vi "Image Viewer.vi"(9 "Stop":bool, 10 "List of Image Files":i32(listbox), 11 "Folder Path":path) -> (2 "2D Picture":picture, 3 "Message BOX":string)   [LabVIEW 2020]
doc: "This VI will load user selected folder containing Image files and will display the selected image on the 2D Picture Display."
uses:
  <vilib>/picture/picture.llb/imagedata.ctl
  <vilib>/Utility/miscctls.llb/LVBoundsTypeDef.ctl
panel:
  in  "OK":bool
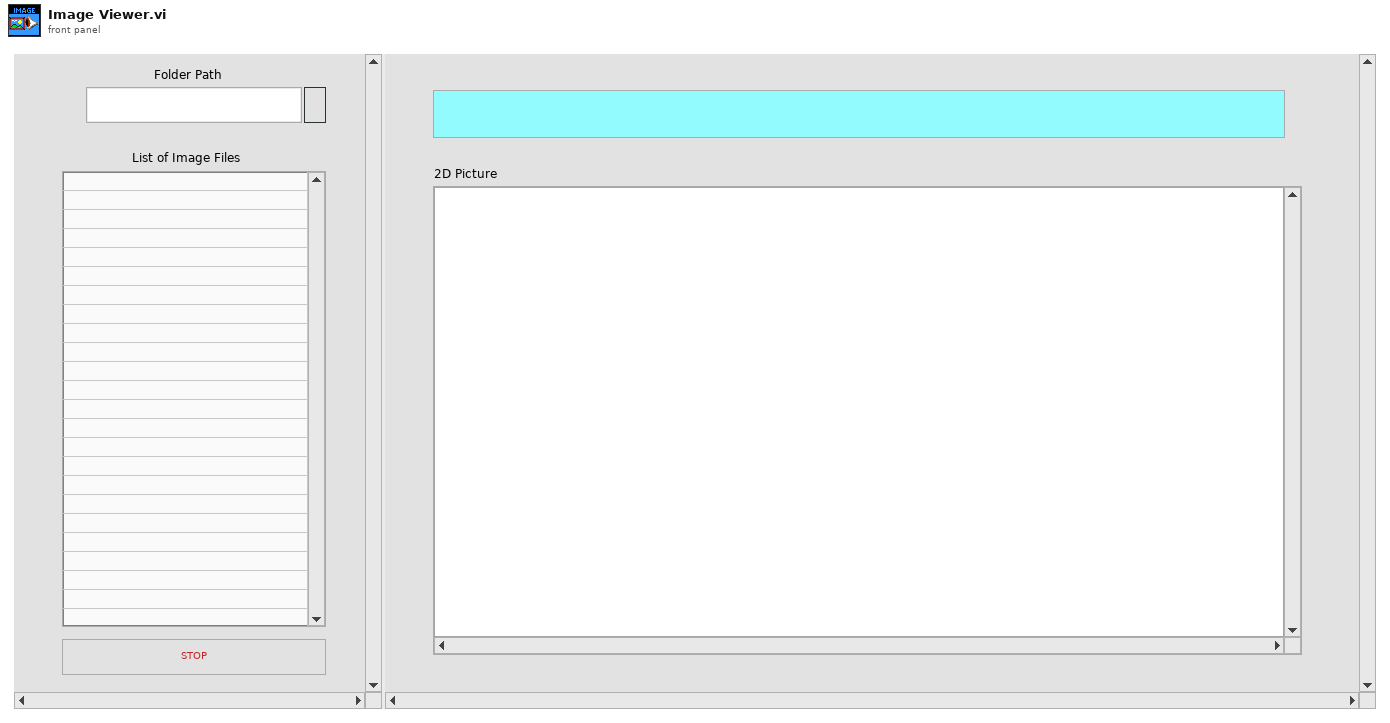
[diagram p1: front panel]
types:
  T1 = enum32{"Invalid", "Standard", "Closed", "Hidden", "Minimized", "Maximized"}
  T2 = enum32{"invalid app kind", "Development System", "Run Time System", "Student Edition", "Embedded LabVIEW", "Evaluation", "Custom"}
  T3 = typedef "LVBoundsTypeDef.ctl" = cluster{"Width":u32, "Height":u32}
  T4 = typedef "imagedata.ctl" = cluster{"image type":i32, "image depth":i32, "image":u8[], "mask":u8[], "colors":u32[], "Rectangle":cluster{"left":i16, "top":i16, "right":i16, "bottom":i16}}
  T5 = cluster{"Core":cluster{"Current VI Reference":refnum<vi>, "Close Panel on Exit?":bool}, "Your Boolean data":bool, "Message BOX":string, "Folder Path":path, "File Name":string, " picture":picture, "image data":T4}
  T6 = cluster{"Current VI Reference":refnum<vi>, "Close Panel on Exit?":bool}
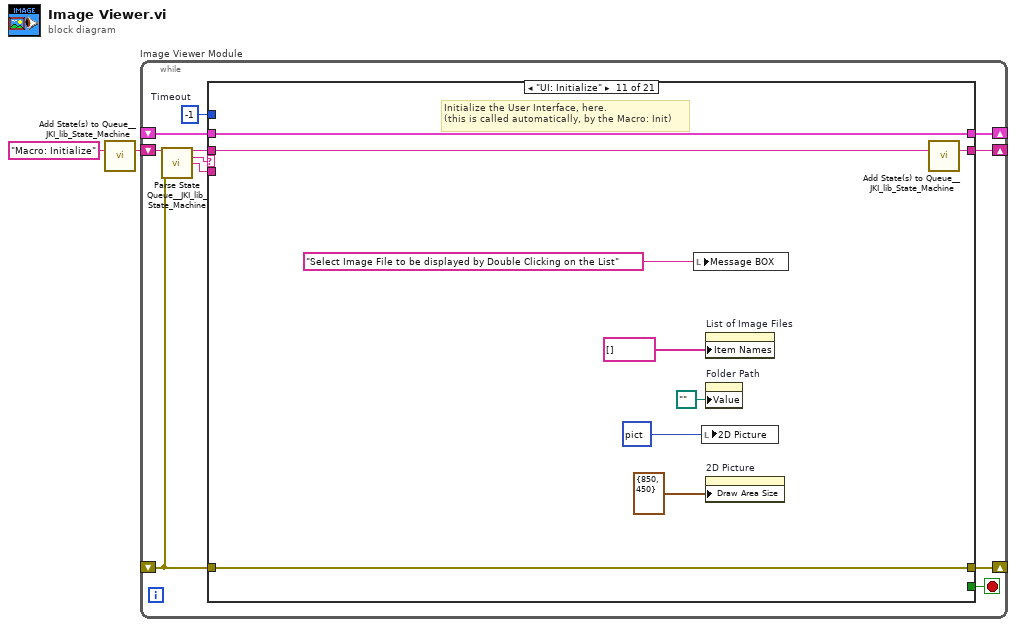
[diagram p0: block diagram]
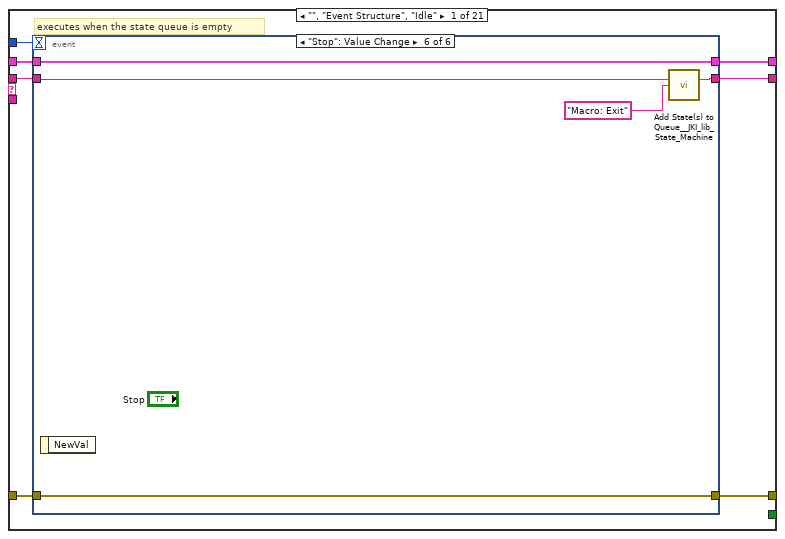
[diagram p2: hidden frame]
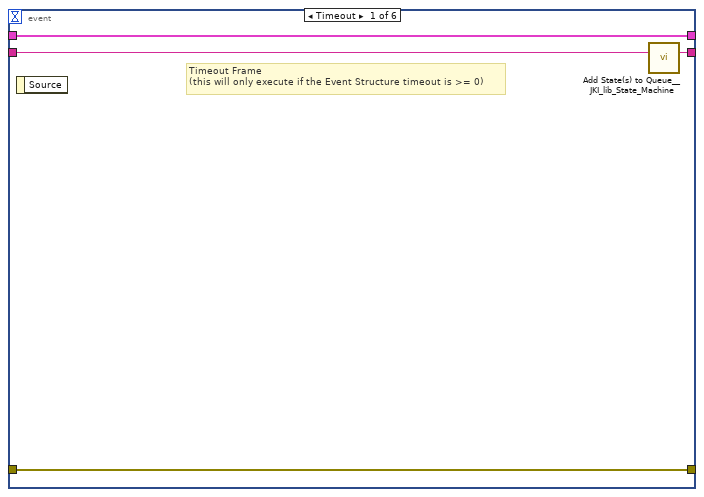
[diagram p3: hidden frame]
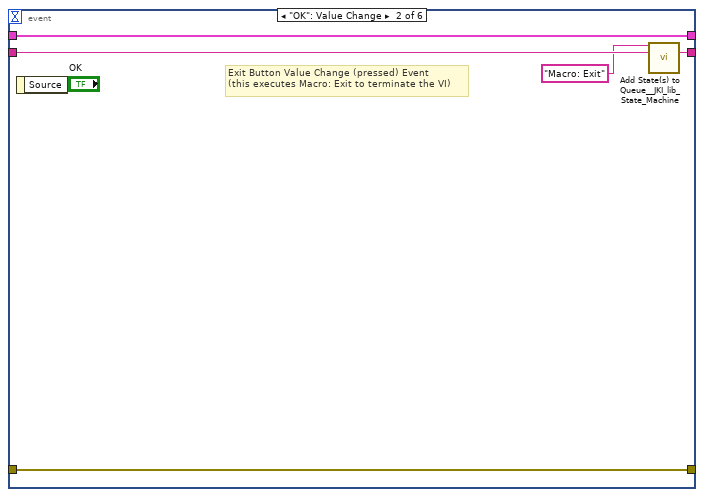
[diagram p4: hidden frame]
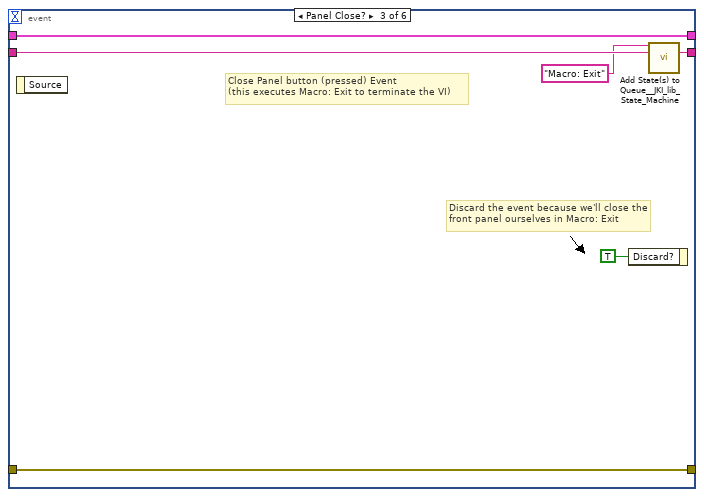
[diagram p5: hidden frame]
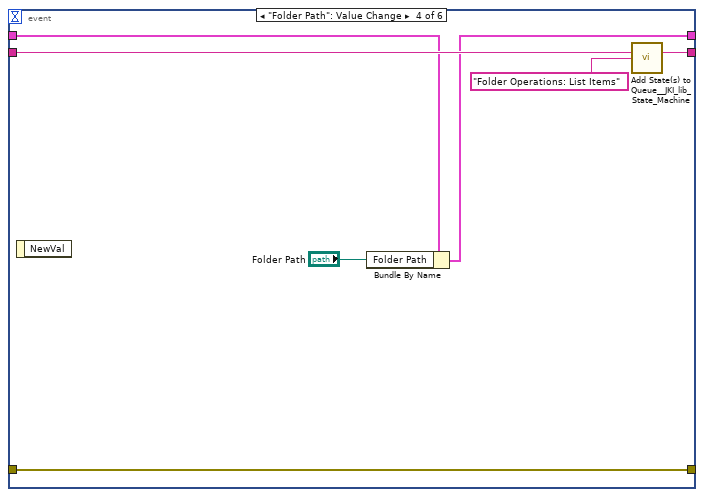
[diagram p6: hidden frame]
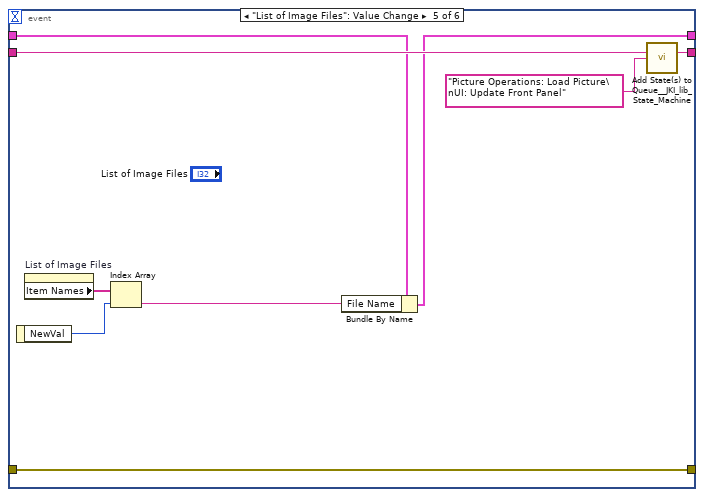
[diagram p7: hidden frame]
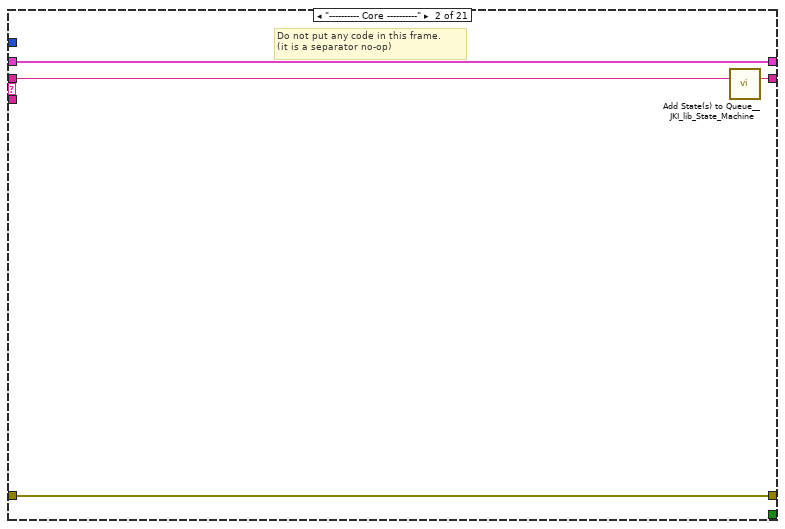
[diagram p8: hidden frame]
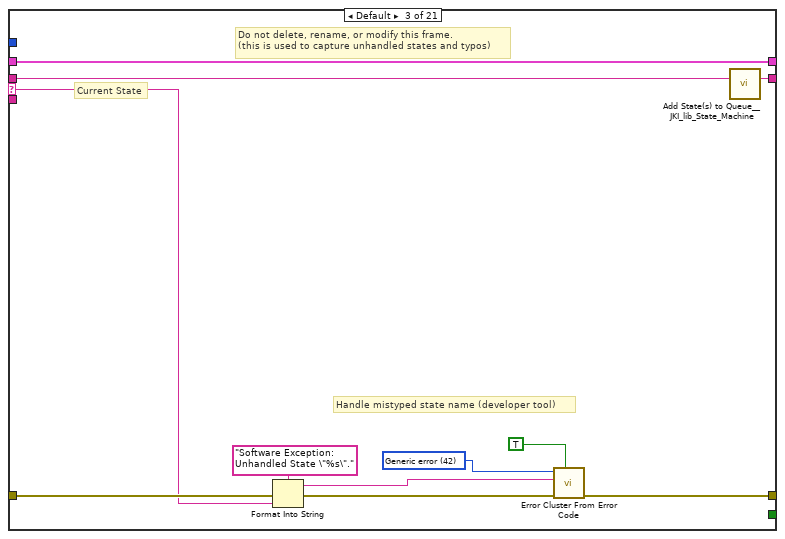
[diagram p9: hidden frame]
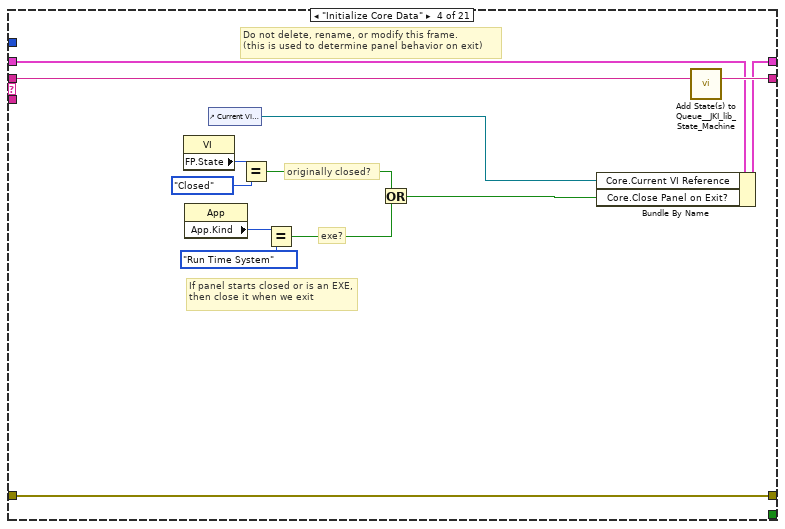
[diagram p10: hidden frame]
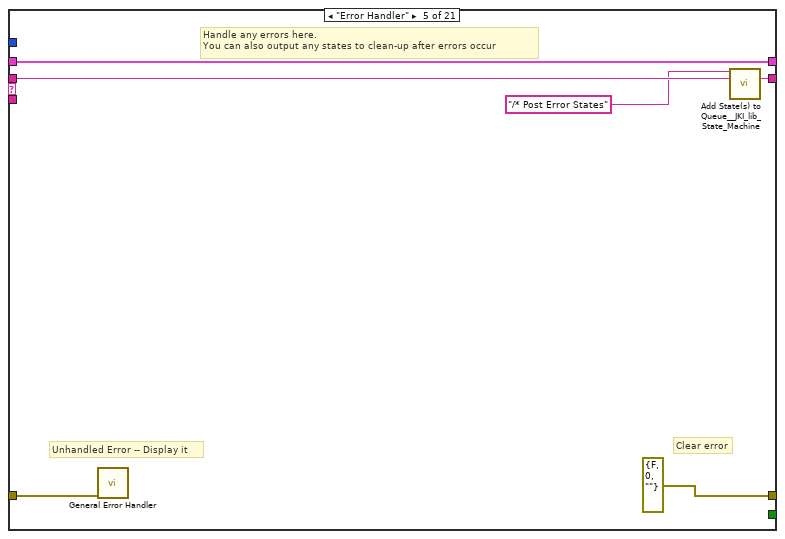
[diagram p11: hidden frame]
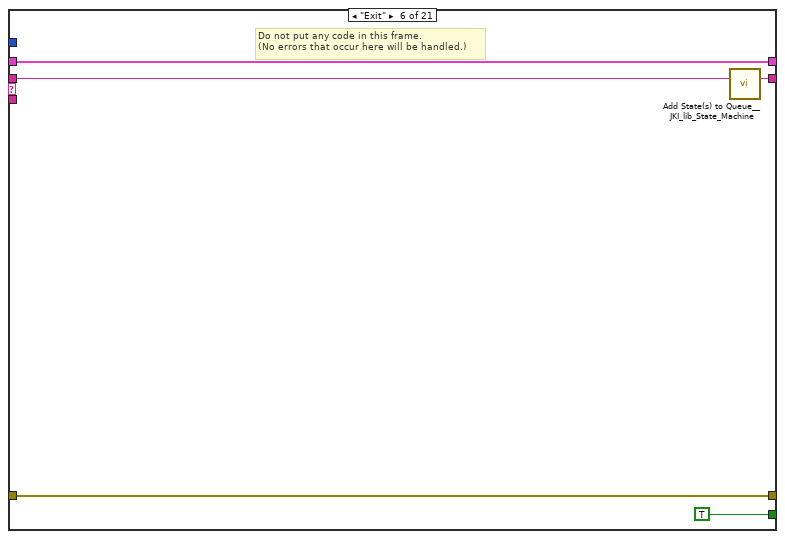
[diagram p12: hidden frame]
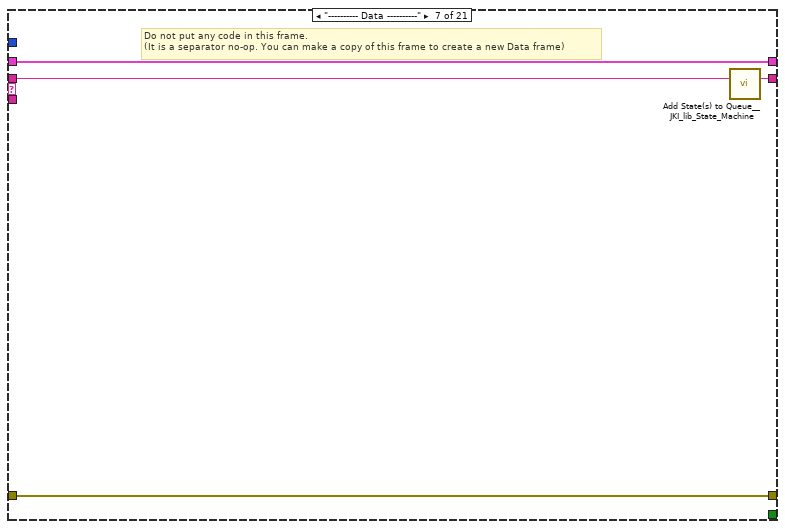
[diagram p13: hidden frame]
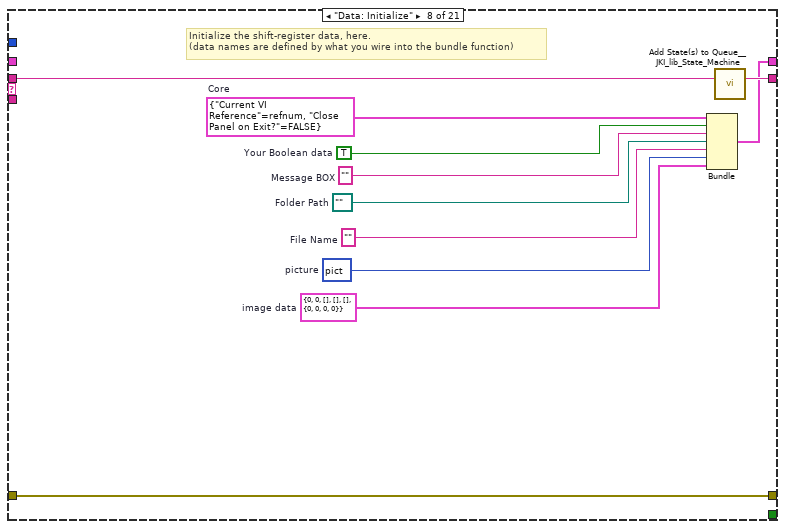
[diagram p14: hidden frame]
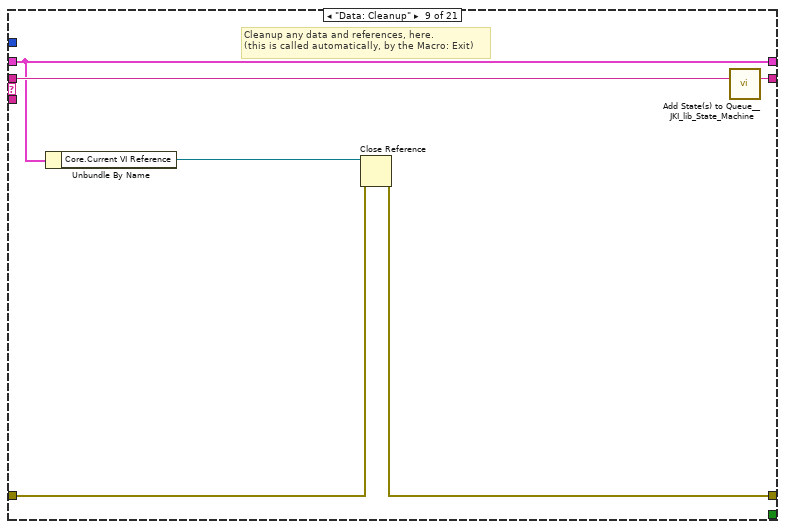
[diagram p15: hidden frame]
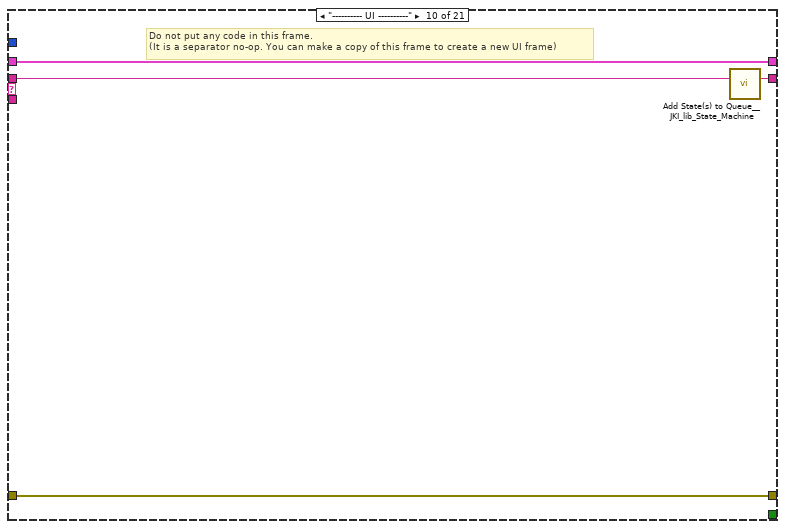
[diagram p16: hidden frame]
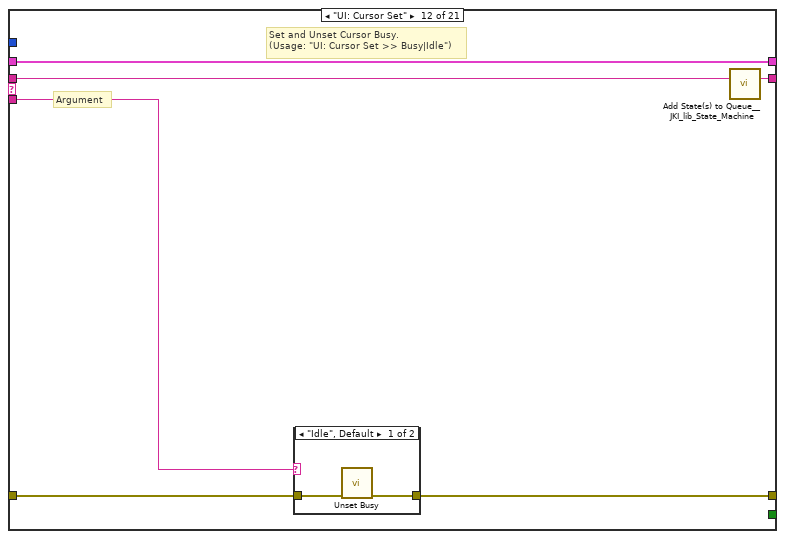
[diagram p17: hidden frame]
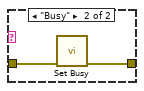
[diagram p18: hidden frame]
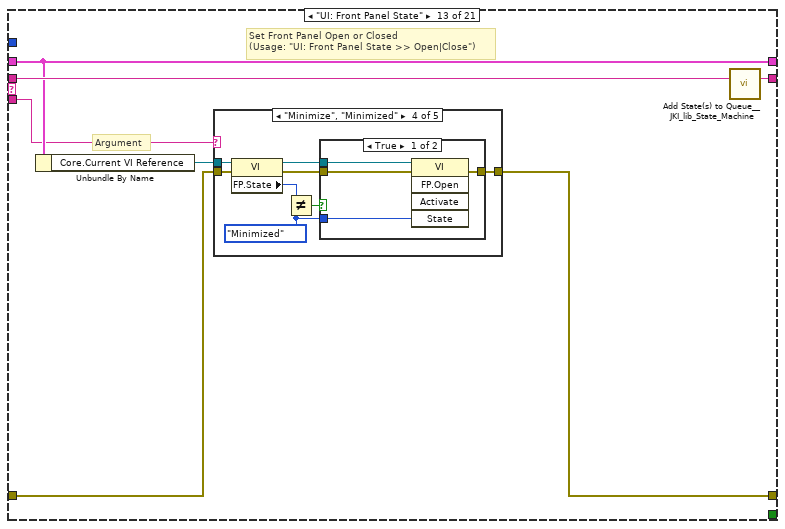
[diagram p19: hidden frame]
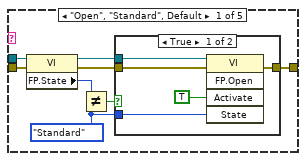
[diagram p20: hidden frame]
diagram:
  n1 = call <vilib>:"Add State(s) to Queue__JKI_lib_State_Machine.vi"("State(s) in (\"\")"="Macro: Initialize") -> ("States Out"=w2:string)  [unwired: 14 in]
  n2 = while "Image Viewer Module" {
    shift-right: [w6] -> _
    shift-left: _ -> [w5]
    shift-right: [w9] -> _
    shift-left: _ -> [w3]
    shift-right: [w8] -> _
    shift-left: w2 -> [w10]
    stop <- w7 stop-if-true
    w4 = -1  # Timeout
    n3 = call <vilib>:"Parse State Queue__JKI_lib_State_Machine.vi"("State Queue"=w10, "Error In (no error)"=w3) -> ("Remaining States"=w12:string, "Current State"=w13:string, "Arguments"=w11:string)  [unwired: 11 in]
    n4 = case shown="\"UI: Initialize\"" w13 {
      selector: w13 -> [_ _ w61 _ _ _ _ _ _ _ _ _ _ _ _ _ _ _ _ _ _]
      tunnel: w12 -> [w20 w60 w65 w84 w90 w95 w99 w110 w116 w120 w129 w135 w146 w224 w228 w233 w243 w247 w253 w257 w274]
      tunnel: w11 -> [_ _ _ _ _ _ _ _ _ _ _ w130 w140 _ _ _ _ _ _ _ _]
      tunnel: w5 -> [w18 w57 w63 w77 w87 w93 w96 _ w111 w117 w127 w133 w142 w221 w225 w230 w240 w244 w250 w254 w268]
      tunnel: [w17 w58 w67 w81 errorcluster {"status"=FALSE, "code"=0, "source"=""} ("error out") w92 w97 w107 w112 w118 w126 w131 w143 w222 w226 w231 w241 w245 w251 w255 w272] -> w9
      tunnel: w3 -> [w16 w58 w66 w81 w86 w92 w97 w107 w113 w118 w126 w132 w144 w222 w226 w231 w241 w245 w251 w255 w272]
      tunnel: [w19 w59 w64 w83 w89 w94 w98 w109 w115 w119 w128 w134 w145 w223 w227 w232 w242 w246 w252 w256 w273] -> w8
      tunnel: [_ _ _ _ _ TRUE _ _ _ _ _ _ _ _ _ _ _ _ _ _ _] -> w7
      tunnel: [w15 w57 w63 w82 w87 w93 w96 w108 w111 w117 w127 w133 w142 w221 w225 w230 w240 w244 w250 w254 w267] -> w6
      tunnel: w4 -> [w14 _ _ _ _ _ _ _ _ _ _ _ _ _ _ _ _ _ _ _ _]
      frame "", "Event Structure", "Idle" {
        # "executes when the state queue is empty"
        n5 = event shown="[5] \"Stop\": Value Change" {
          selector: _ -> [_ _ _ _ _ _]
          dyn-events: _ -> [_ _ _ _ _ _]
          timeout: w14 -> [_ _ _ _ _ _]
          tunnel: w20 -> [w24 w29 w35 w41 w50 w54]
          tunnel: [w23 w28 w34 w42 w51 w55] -> w19
          tunnel: w18 -> [w21 w26 w32 w40 w46 w53]
          tunnel: [w22 w27 w33 w36 w49 w56] -> w17
          tunnel: w16 -> [w22 w27 w33 w36 w49 w56]
          tunnel: [w21 w26 w32 w39 w45 w53] -> w15
          event Timeout {
            # "Timeout Frame\n(this will only execute if the Event Structure timeout is >= 0)"
            n6 = event-data() -> ()  [unwired: 1 in, 1 out]
            n7 = call <vilib>:"Add State(s) to Queue__JKI_lib_State_Machine.vi"("State(s) in (\"\")"=w24) -> ("States Out"=w23:string)  [unwired: 14 in]
          }
          event "OK": Value Change {
            # "Exit Button Value Change (pressed) Event\n(this executes Macro: Exit to terminate the VI)"
            n8 = event-data() -> ()  [unwired: 1 in, 1 out]
            n9 = call <vilib>:"Add State(s) to Queue__JKI_lib_State_Machine.vi"("State(s) in Front (\"\")"="Macro: Exit", "State(s) in (\"\")"=w29) -> ("States Out"=w28:string)  [unwired: 13 in]
          }
          event Panel Close? {
            # "Discard the event because we'll close the front panel ourselves in Macro: Exit"
            # "Close Panel button (pressed) Event\n(this executes Macro: Exit to terminate the VI)"
            n10 = event-data() -> ()  [unwired: 1 in, 1 out]
            n11 = event-data("Discard?"=TRUE) -> ()  [unwired: 1 in, 1 out]
            n12 = call <vilib>:"Add State(s) to Queue__JKI_lib_State_Machine.vi"("State(s) in Front (\"\")"="Macro: Exit", "State(s) in (\"\")"=w35) -> ("States Out"=w34:string)  [unwired: 13 in]
          }
          event "Folder Path": Value Change {
            n13 = event-data() -> ()  [unwired: 1 in, 1 out]
            n14 = Bundle By Name(cluster=w40, "Folder Path"="Folder Path") -> (w39:T5)
            n15 = call <vilib>:"Add State(s) to Queue__JKI_lib_State_Machine.vi"("State(s) in (\"\")"=w41, "State(s) at Back (\"\")"="Folder Operations: List Items" ("State(s) at Back (\"\")")) -> ("States Out"=w42:string)  [unwired: 13 in]
          }
          event "List of Image Files": Value Change {
            n16 = event-data() -> ("NewVal"=w47:i32)  [unwired: 1 in]
            n17 = property on="List of Image Files" class="LstBox (strict)"() -> ("Item Names"=w48:string[])  [unwired: 2 in, 2 out]
            n18 = Index Array(array=w48, index=w47) -> (element=w44:string)
            n19 = Bundle By Name(cluster=w46, "File Name"=w44) -> (w45:T5)
            n20 = call <vilib>:"Add State(s) to Queue__JKI_lib_State_Machine.vi"("State(s) in (\"\")"=w50, "State(s) at Back (\"\")"="Picture Operations: Load Picture\nUI: Update Front Panel" ("State(s) at Back (\"\")")) -> ("States Out"=w51:string)  [unwired: 13 in]
          }
          event "Stop": Value Change {
            n21 = event-data() -> ()  [unwired: 1 in, 1 out]
            n22 = call <vilib>:"Add State(s) to Queue__JKI_lib_State_Machine.vi"("State(s) in (\"\")"=w54, "State(s) at Back (\"\")"="Macro: Exit") -> ("States Out"=w55:string)  [unwired: 13 in]
          }
        }
      }
      frame "---------- Core ----------" {
        # "Do not put any code in this frame.\n(it is a separator no-op)"
        n23 = call <vilib>:"Add State(s) to Queue__JKI_lib_State_Machine.vi"("State(s) in (\"\")"=w60) -> ("States Out"=w59:string)  [unwired: 14 in]
      }
      frame Default {
        w70 = 42 items=["No error", "Argument error", "Memory is full", "Out of zone", "End of file", "File already open", "Generic file I/O error", "File not found", "File permission error", "Disk is full", "Duplicate path", "Too many files open", "System feature not enabled", "Resource file not found", "Cannot add resource", "Resource not found", "Image not found", "Image memory error", "Pen does not exist", "Config type invalid", "Config token not found", "Config parse error", "Config memory error", "Bad external code format", "Bad external code offset", "External code not present", "Null window", "Destroy window error", "Null menu", "Print aborted", "Bad print record", "Print driver error", "Windows error during printing", "Memory error during printing", "Print dialog error", "Generic print error", "Invalid device refnum", "Device not found", "Device parameter error", "Device unit error", "Cannot open device", "Device call aborted", "Generic error", "Cancelled by user", "Object ID too low", "Object ID too high", "Object not in heap", "Unknown heap", "Unknown object (invalid DefProc)", "Unknown object (DefProc not in table)", "Message out of range", "Invalid (null) method", "Unknown message", "Manager call not supported", "Bad address", "Network operation in progress", "Network operation timed out", "Connection is busy", "Network attribute not supported", "Network error", "Address in use", "System out of memory", "Connection aborted", "Connection refused", "Not connected", "Already connected", "Connection closed", "Initialization error (interapplication manager)", "Bad occurrence", "Wait on unbound occurrence handler", "Occurrence queue overflow", "Datalog type conflict", "Unused", "Unrecognized type (interapplication manager)", "Memory corrupt", "Failed to make temporary DLL", "Old CIN version", "Drag socket not found", "Failed to load drop-object", "Failed to register OLE object", "Failed to release OLE object", "Format specifier type mismatch", "Unknown format specifier", "Too few format specifiers", "Too many format specifiers", "Scan failed", "Newer CIN version", "Error converting to variant", "Runtime menu error", "Password tampered", "Variant attribute not found", "Incompatible variant data type", "Event data is not available", "Event Store is not present", "Occurrence is not found", "Event Queue is not created", "Event info is not available", "Refnum passed is NULL", "Error retrieving Class GUID", "Error retrieving CoClass GUID", "Error retrieving TypeLib GUID.", "Bad built application magic bytes.", "Specific driver is different from the specific driver associated with the Logical Name.", "There is no session opened to the class driver.", "Max Error", "MAX - Error with config objects", "MAX - Error loading configuration", "MAX - Group not supported"]
        # "Current State"
        # "Do not delete, rename, or modify this frame.\n(this is used to capture unhandled states and typos)"
        # "Handle mistyped state name (developer tool)"
        n24 = Format Into String(format string="Software Exception: Unhandled State \"%s\"." ("message"), error in=w66, w61) -> (resulting string=w69:string, error out=w68:errorcluster)  [unwired: 1 in]
        n25 = call <vilib>:"Error Cluster From Error Code.vi"("show call chain? (False)"=TRUE, "error in (no error)"=w68, "error message (\"\")"=w69, "error code (0)"=w70) -> ("error out"=w67:errorcluster)  [unwired: 5 in]
        n26 = call <vilib>:"Add State(s) to Queue__JKI_lib_State_Machine.vi"("State(s) in (\"\")"=w65) -> ("States Out"=w64:string)  [unwired: 14 in]
      }
      frame "Initialize Core Data" {
        # "Do not delete, rename, or modify this frame.\n(this is used to determine panel behavior on exit)"
        # "originally closed?"
        # "exe?"
        # "If panel starts closed or is an EXE, then close it when we exit"
        n27 = property class="VI"() -> ("FP.State"=w74:T1)  [unwired: 2 in, 2 out]
        n28 = property class="App"() -> ("App.Kind"=w80:T2)  [unwired: 2 in, 2 out]
        n29 = control-ref of="Current VI Reference"() -> (w75:refnum<vi>)
        n30 = Equal?(x=w74, y=T1."Closed" ("Front Panel Window:State")) -> (x = y?=w72:bool)
        n31 = Equal?(x=w80, y=T2."Run Time System" ("Application:Kind")) -> (x = y?=w78:bool)
        n32 = Or(x=w72, y=w78) -> (x .or. y?=w76:bool)
        n33 = Bundle By Name(cluster=w77, "Core.Current VI Reference"=w75, "Core.Close Panel on Exit?"=w76) -> (w82:T5)
        n34 = call <vilib>:"Add State(s) to Queue__JKI_lib_State_Machine.vi"("State(s) in (\"\")"=w84) -> ("States Out"=w83:string)  [unwired: 14 in]
      }
      frame "Error Handler" {
        # "Unhandled Error -- Display it"
        # "Handle any errors here.\nYou can also output any states to clean-up after errors occur"
        # "Clear error"
        n35 = call <vilib>:"General Error Handler.vi"("error in (no error)"=w86) -> ()  [unwired: 10 in, 5 out]
        n36 = call <vilib>:"Add State(s) to Queue__JKI_lib_State_Machine.vi"("State(s) in Front (\"\")"="/* Post Error States", "State(s) in (\"\")"=w90) -> ("States Out"=w89:string)  [unwired: 13 in]
      }
      frame "Exit" {
        # "Do not put any code in this frame.\n(No errors that occur here will be handled.)"
        n37 = call <vilib>:"Add State(s) to Queue__JKI_lib_State_Machine.vi"("State(s) in (\"\")"=w95) -> ("States Out"=w94:string)  [unwired: 14 in]
      }
      frame "---------- Data ----------" {
        # "Do not put any code in this frame.\n(It is a separator no-op. You can make a copy of this frame to create a new Data frame)"
        n38 = call <vilib>:"Add State(s) to Queue__JKI_lib_State_Machine.vi"("State(s) in (\"\")"=w99) -> ("States Out"=w98:string)  [unwired: 14 in]
      }
      frame "Data: Initialize" {
        w100 = T4 {"image type"=0, "image depth"=0, "image"=[], "mask"=[], "colors"=[], "Rectangle"={"left"=0, "top"=0, "right"=0, "bottom"=0}}  # image data
        w101 = picture data[5B]  # picture
        w102 = ""  # File Name
        w103 = path ""  # Folder Path
        w104 = T6 {"Current VI Reference"=refnum, "Close Panel on Exit?"=FALSE}  # Core
        w106 = TRUE  # Your Boolean data
        w105 = ""  # Message BOX
        # "Initialize the shift-register data, here.\n(data names are defined by what you wire into the bundle function)"
        n39 = Bundle("Core"=w104, "Your Boolean data"=w106, "Message BOX"=w105, "Folder Path"=w103, "File Name"=w102, "picture"=w101, "image data"=w100) -> (w108:T5)  [unwired: 1 in]
        n40 = call <vilib>:"Add State(s) to Queue__JKI_lib_State_Machine.vi"("State(s) in (\"\")"=w110) -> ("States Out"=w109:string)  [unwired: 14 in]
      }
      frame "Data: Cleanup" {
        # "Cleanup any data and references, here.\n(this is called automatically, by the Macro: Exit)"
        n41 = Unbundle By Name(w111) -> ("Core.Current VI Reference"=w114:refnum<vi>)
        n42 = Close Reference(reference=w114, error in (no error)=w113) -> (error out=w112:errorcluster)
        n43 = call <vilib>:"Add State(s) to Queue__JKI_lib_State_Machine.vi"("State(s) in (\"\")"=w116) -> ("States Out"=w115:string)  [unwired: 14 in]
      }
      frame "---------- UI ----------" {
        # "Do not put any code in this frame.\n(It is a separator no-op. You can make a copy of this frame to create a new UI frame)"
        n44 = call <vilib>:"Add State(s) to Queue__JKI_lib_State_Machine.vi"("State(s) in (\"\")"=w120) -> ("States Out"=w119:string)  [unwired: 14 in]
      }
      frame "UI: Initialize" {
        # "Initialize the User Interface, here.\n(this is called automatically, by the Macro: Init)"
        n45 = local write "Message BOX"("Select Image File to be displayed by Double Clicking on the List" ("Message BOX")) -> ()
        n46 = local write "2D Picture"(picture data[5B] ("2D Picture")) -> ()
        n47 = property on="List of Image Files" class="LstBox (strict)"("Item Names"=string[] []) -> ()  [unwired: 2 in, 2 out]
        n48 = property on="Folder Path" class="Path"("Value"=path "" ("Folder Path")) -> ()  [unwired: 2 in, 2 out]
        n49 = property on="2D Picture" class="Pict"("Draw Area Size"=T3 {"Width"=850, "Height"=450}) -> ()  [unwired: 2 in, 2 out]
        n50 = call <vilib>:"Add State(s) to Queue__JKI_lib_State_Machine.vi"("State(s) in (\"\")"=w129) -> ("States Out"=w128:string)  [unwired: 14 in]
      }
      frame "UI: Cursor Set" {
        # "Argument"
        # "Set and Unset Cursor Busy.\n(Usage: \"UI: Cursor Set >> Busy|Idle\")"
        n51 = case shown="\"Idle\", Default" w130 {
          tunnel: w132 -> [w137 w139]
          tunnel: [w136 w138] -> w131
          frame "Idle", Default {
            n52 = call <vilib>:"Unset Busy.vi"("error in (no error)"=w137) -> ("error out"=w136:errorcluster)  [unwired: 10 in]
          }
          frame "Busy" {
            n53 = call <vilib>:"Set Busy.vi"("error in (no error)"=w139) -> ("error out"=w138:errorcluster)  [unwired: 9 in, 1 out]
          }
        }
        n54 = call <vilib>:"Add State(s) to Queue__JKI_lib_State_Machine.vi"("State(s) in (\"\")"=w135) -> ("States Out"=w134:string)  [unwired: 14 in]
      }
      frame "UI: Front Panel State" {
        # "Argument"
        # "Set Front Panel Open or Closed\n(Usage: \"UI: Front Panel State >> Open|Close\")"
        n55 = Unbundle By Name(w142) -> ("Core.Current VI Reference"=w141:refnum<vi>)
        n56 = case shown="\"Minimize\", \"Minimized\"" w140 {
          tunnel: w144 -> [w152 w167 w178 w191 w204]
          tunnel: [w154 w168 w180 w193 w206] -> w143
          tunnel: w141 -> [w153 w165 w179 w192 w205]
          frame "Open", "Standard", Default {
            w147 = T1."Standard" ("State")
            n57 = property class="VI"(reference=w153, error in=w152) -> (reference out=w150:refnum<vi>, error out=w151:errorcluster, "FP.State"=w149:T1)
            n58 = Not Equal?(x=w149, y=w147) -> (x != y?=w148:bool)
            n59 = case shown="True" w148 {
              tunnel: [w158 w160] -> w154
              tunnel: w151 -> [w157 w160]
              tunnel: w150 -> [w156 _]
              tunnel: w147 -> [w155 _]
              frame True {
                n60 = invoke class="VI" method="FP.Open"(reference=w156, error in=w157, "Activate"=TRUE, "State"=w155) -> (error out=w158:errorcluster)  [unwired: 1 in, 4 out]
              }
              frame False {
              }
            }
          }
          frame "Close", "Closed" {
            n61 = property class="VI"(reference=w165, error in=w167) -> (reference out=w164:refnum<vi>, error out=w166:errorcluster, "FP.State"=w162:T1)
            n62 = Not Equal?(x=w162, y=T1."Closed" ("Front Panel Window:State")) -> (x != y?=w161:bool)
            n63 = case shown="True" w161 {
              tunnel: [w169 w172] -> w168
              tunnel: w166 -> [w169 w171]
              tunnel: w164 -> [_ w170]
              frame False {
              }
              frame True {
                n64 = invoke class="VI" method="FP.Close"(reference=w170, error in=w171) -> (error out=w172:errorcluster)  [unwired: 1 in, 2 out]
              }
            }
          }
          frame "Hidden", "Hide" {
            w173 = T1."Hidden" ("State")
            n65 = property class="VI"(reference=w179, error in=w178) -> (reference out=w176:refnum<vi>, error out=w177:errorcluster, "FP.State"=w175:T1)
            n66 = Not Equal?(x=w175, y=w173) -> (x != y?=w174:bool)
            n67 = case shown="True" w174 {
              tunnel: [w184 w185] -> w180
              tunnel: w177 -> [w183 w185]
              tunnel: w176 -> [w182 _]
              tunnel: w173 -> [w181 _]
              frame True {
                n68 = invoke class="VI" method="FP.Open"(reference=w182, error in=w183, "State"=w181) -> (error out=w184:errorcluster)  [unwired: 2 in, 4 out]
              }
              frame False {
              }
            }
          }
          frame "Minimize", "Minimized" {
            w186 = T1."Minimized" ("State")
            n69 = property class="VI"(reference=w192, error in=w191) -> (reference out=w189:refnum<vi>, error out=w190:errorcluster, "FP.State"=w188:T1)
            n70 = Not Equal?(x=w188, y=w186) -> (x != y?=w187:bool)
            n71 = case shown="True" w187 {
              tunnel: [w197 w198] -> w193
              tunnel: w190 -> [w196 w198]
              tunnel: w189 -> [w195 _]
              tunnel: w186 -> [w194 _]
              frame True {
                n72 = invoke class="VI" method="FP.Open"(reference=w195, error in=w196, "State"=w194) -> (error out=w197:errorcluster)  [unwired: 2 in, 4 out]
              }
              frame False {
              }
            }
          }
          frame "Maximize", "Maximized" {
            w199 = T1."Maximized" ("State")
            n73 = property class="VI"(reference=w205, error in=w204) -> (reference out=w202:refnum<vi>, error out=w203:errorcluster, "FP.State"=w201:T1)
            n74 = Not Equal?(x=w201, y=w199) -> (x != y?=w200:bool)
            n75 = case shown="True" w200 {
              tunnel: [w210 w211] -> w206
              tunnel: w203 -> [w209 w211]
              tunnel: w202 -> [w208 _]
              tunnel: w199 -> [w207 _]
              frame True {
                n76 = invoke class="VI" method="FP.Open"(reference=w208, error in=w209, "State"=w207) -> (error out=w210:errorcluster)  [unwired: 2 in, 4 out]
              }
              frame False {
              }
            }
          }
        }
        n77 = call <vilib>:"Add State(s) to Queue__JKI_lib_State_Machine.vi"("State(s) in (\"\")"=w146) -> ("States Out"=w145:string)  [unwired: 14 in]
      }
      frame "UI: Update Front Panel" {
        # "Front Panel update based on USER input\n(Updates Front Panel 2D Picture Box with the Image)"
        n78 = Unbundle By Name(w221) -> ("File Name"=w220:string, "image data"=w217:T4, "picture"=→"2D Picture":picture)
        n79 = Concatenate Strings("You have Selected " ("string"), w220) -> (→"Message BOX":string)
        n80 = Unbundle By Name(w217) -> ("Rectangle.right"=w216:i16, "Rectangle.bottom"=w215:i16)
        n81 = Bundle(cluster=cluster{"right":i16, "bottom":i16} {"right"=0, "bottom"=0}, "right"=w216, "bottom"=w215) -> (w213:cluster{"right":i16, "bottom":i16})
        n82 = property on="2D Picture" class="Pict"("Draw Area Size"=w213) -> ()  [unwired: 2 in, 2 out]
        n83 = call <vilib>:"Add State(s) to Queue__JKI_lib_State_Machine.vi"("State(s) in (\"\")"=w224) -> ("States Out"=w223:string)  [unwired: 14 in]
      }
      frame "---------- Macro ----------" {
        # "Do not put any code in this frame.\n(It is a separator no-op. You can make a copy of this frame to create a new Macro frame)"
        n84 = call <vilib>:"Add State(s) to Queue__JKI_lib_State_Machine.vi"("State(s) in (\"\")"=w228) -> ("States Out"=w227:string)  [unwired: 14 in]
      }
      frame "Macro: Initialize" {
        w229 = "Data: Initialize\nInitialize Core Data\nUI: Initialize\nUI: Front Panel State >> Open"  # Data: Initialize Initialize Core Data UI: Initialize UI: Front Panel State >> Open
        # "Initialization Macro\n(This is called once, when the VI starts)"
        n85 = call <vilib>:"Add State(s) to Queue__JKI_lib_State_Machine.vi"("State(s) in Front (\"\")"=w229, "State(s) in (\"\")"=w233) -> ("States Out"=w232:string)  [unwired: 13 in]
      }
      frame "Macro: Exit" {
        # "Exit Macro\n(This is called once, when the VI exits)"
        n86 = Unbundle By Name(w240) -> ("Core.Close Panel on Exit?"=w239:bool)
        n87 = Select(t="UI: Front Panel State >> Close", s=w239, f="") -> (s? t:f=w236:string)
        n88 = call <vilib>:"Add State(s) to Queue__JKI_lib_State_Machine.vi"("State(s) in (\"\")"=w236, "State(s) at Back (\"\")"="Data: Cleanup\nExit") -> ("States Out"=w234:string)  [unwired: 13 in]
        n89 = call <vilib>:"Add State(s) to Queue__JKI_lib_State_Machine.vi"("State(s) in Front (\"\")"=w234, "State(s) in (\"\")"=w243) -> ("States Out"=w242:string)  [unwired: 13 in]
      }
      frame "---------- Folder Operations ----------" {
        # "Template Separator\n(You can make a copy of, or modify, this frame)"
        n90 = call <vilib>:"Add State(s) to Queue__JKI_lib_State_Machine.vi"("State(s) in (\"\")"=w247) -> ("States Out"=w246:string)  [unwired: 14 in]
      }
      frame "Folder Operations: List Items" {
        # "List FOLDER Content\n(Selected Folder content is listed and updated on the front Panel)"
        n91 = Unbundle By Name(w250) -> ("Folder Path"=w249:path)
        n92 = List Folder(path=w249) -> (filenames=w248:string[])  [unwired: 3 in, 3 out]
        n93 = property on="List of Image Files" class="LstBox (strict)"("Item Names"=w248) -> ()  [unwired: 2 in, 2 out]
        n94 = call <vilib>:"Add State(s) to Queue__JKI_lib_State_Machine.vi"("State(s) in (\"\")"=w253) -> ("States Out"=w252:string)  [unwired: 14 in]
      }
      frame "---------- Picture Operations ----------" {
        # "Template Separator\n(You can make a copy of, or modify, this frame)"
        n95 = call <vilib>:"Add State(s) to Queue__JKI_lib_State_Machine.vi"("State(s) in (\"\")"=w257) -> ("States Out"=w256:string)  [unwired: 14 in]
      }
      frame "Picture Operations: Load Picture" {
        # "Loads Picture from selected Folder Path\n(Loads the Selected picture into the Front Panel window)"
        n96 = Unbundle By Name(w268) -> ("Folder Path"=w271:path, "File Name"=w264:string)
        n97 = Path To String(path=w271) -> (string=w270:string)
        n98 = Concatenate Strings(w270, "\\" ("string"), w264) -> (w265:string)
        n99 = Build Path(name or relative path=w265) -> (appended path=w261:path)  [unwired: 1 in]
        n100 = call <vilib>:"Get File Extension.vi"("file"=w261) -> ("lowercase file extension"=w263:string, "dup file"=w259:path)  [unwired: 6 in, 3 out]
        n101 = Equal?(x=w263, y="png") -> (x = y?=w260:bool)
        n102 = case shown="False" w260 {
          tunnel: w259 -> [w275 w278]
          tunnel: [w276 w277] -> w258
          frame False {
            n103 = call <vilib>:"Read JPEG File.vi"("path to JPEG file"=w275) -> ("image data"=w276:T4)  [unwired: 8 in, 2 out]
          }
          frame True {
            n104 = call <vilib>:"Read PNG File.vi"("path to PNG file"=w278) -> ("image data"=w277:T4)  [unwired: 8 in, 2 out]
          }
        }
        n105 = call <vilib>:"Draw Flattened Pixmap.vi"("image data"=w258) -> ("new picture"=w266:picture)  [unwired: 8 in]
        n106 = Bundle By Name(cluster=w268, "image data"=w258, "picture"=w266) -> (w267:T5)
        n107 = call <vilib>:"Add State(s) to Queue__JKI_lib_State_Machine.vi"("State(s) in (\"\")"=w274) -> ("States Out"=w273:string)  [unwired: 14 in]
      }
    }
  }
